vi "ConfigurationDialog.vi"(8 "error in":errorcluster, 11 "Configuration Settings In":T1) -> (0 "error out":errorcluster, 3 "Configuration Settings Out":T1)   [LabVIEW 2025]
uses:
  Typedefs/ConfigurationSettings.ctl
panel:
  in  "Plot.Line Style":u8
  in  "Plot.Line Width":u8
  in  "Cancel":bool
  in  "Confirm":bool
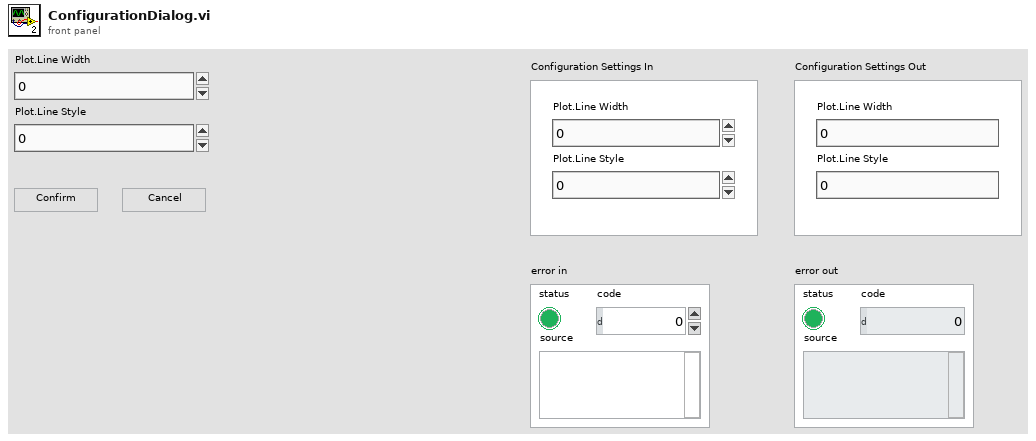
[diagram p1: front panel]
types:
  T1 = typedef "ConfigurationSettings.ctl" = cluster{"Plot.Line Width":u8, "Plot.Line Style":u8}
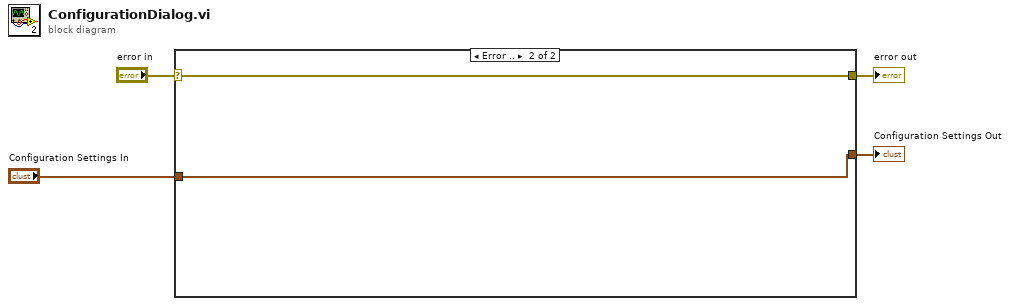
[diagram p0: block diagram]
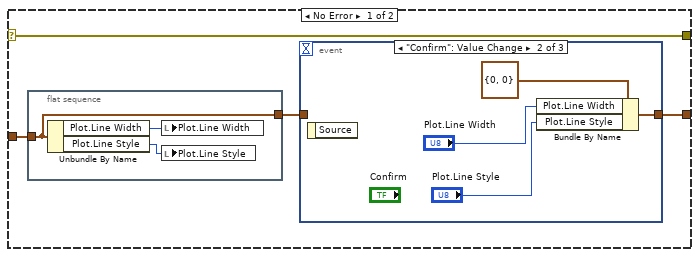
[diagram p2: hidden frame]
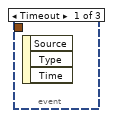
[diagram p3: hidden frame]
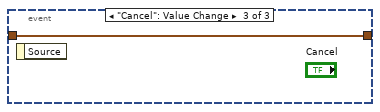
[diagram p4: hidden frame]
diagram:
  n1 = case shown="Error .." "error in" {
    selector: "error in" -> [w8 w18]
    tunnel: [w8 w18] -> w3
    tunnel: "Configuration Settings In" -> [w6 w17]
    tunnel: [w7 w17] -> w1
    frame No Error {
      n2 = flat-sequence {
        tunnel: w6 -> [w9]
        tunnel: [w9] -> w5
        frame #0 {
          n3 = Unbundle By Name(w9) -> ("Plot.Line Width"=w11:u8, "Plot.Line Style"=w10:u8)
          n4 = local write "Plot.Line Width"(w11) -> ()
          n5 = local write "Plot.Line Style"(w10) -> ()
        }
      }
      n6 = event shown="[1] \"Confirm\": Value Change" {
        selector: _ -> [_ _ _]
        dyn-events: _ -> [_ _ _]
        timeout: _ -> [_ _ _]
        tunnel: [_ w12 w16] -> w7
        tunnel: w5 -> [_ _ w16]
        event Timeout {
          n7 = event-data() -> ()  [unwired: 1 in, 3 out]
        }
        event "Confirm": Value Change {
          n8 = event-data() -> ()  [unwired: 1 in, 1 out]
          n9 = Bundle By Name(cluster=T1 {"Plot.Line Width"=0, "Plot.Line Style"=0} ("Configuration Settings Out"), "Plot.Line Width"="Plot.Line Width", "Plot.Line Style"="Plot.Line Style") -> (w12:T1)
        }
        event "Cancel": Value Change {
          n10 = event-data() -> ()  [unwired: 1 in, 1 out]
        }
      }
    }
    frame Error {
    }
  }
  "error out" <- w3
  "Configuration Settings Out" <- w1
